vi "saveFuzzyMap2MCU.vi"(1 "Config":T1, 3 "error in (no error)":errorcluster) -> (10 "error out":errorcluster)   [LabVIEW 2016]
uses:
  Settings/Settings.ctl
  Logging/Logging Configuration.ctl
  Hardware Configuration.ctl
  <vilib>/NI Modbus.llb/MB Serial Master Query Write Multiple Registers (poly).vi
  Logging/Logging.lvlib
  Acquisition.lvlib
  Settings/Settings.lvlib
panel:
  out "Exception Code":u8 format="%.0x"
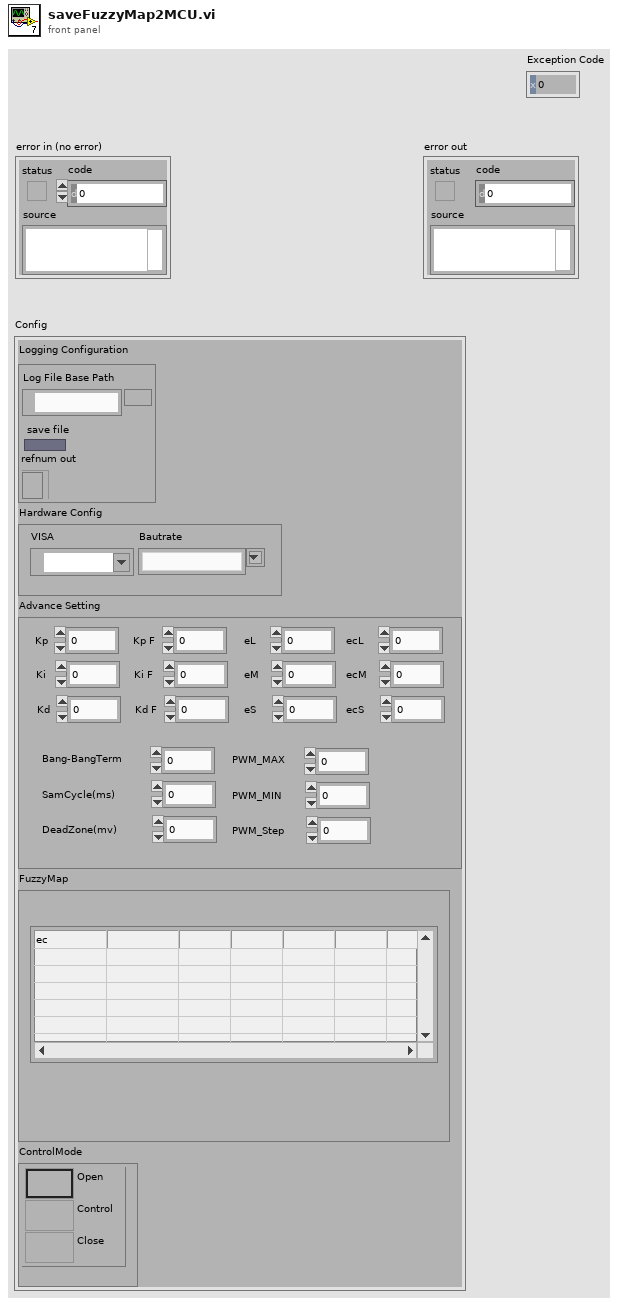
[diagram p1: front panel]
types:
  T1 = typedef "Settings.lvlib/Settings.ctl" = cluster{"Logging Configuration":T2, "Hardware Config":cluster{"Bautrate":string, "VISA":T3}, "Advance Setting":cluster{"PWM_Step":dbl, "PWM_MIN":dbl, "PWM_MAX":dbl, "DeadZone(mv)":dbl, "SamCycle(ms)":dbl, "Bang-BangTerm":dbl, "ecS":dbl, "ecM":dbl, "ecL":dbl, "eS":dbl, "eM":dbl, "eL":dbl, "Kd F":dbl, "Ki F":dbl, "Kp F":dbl, "Kd":dbl, "Ki":dbl, "Kp":dbl}, "FuzzyMap":cluster{"Table":string[][]}, "ControlMode":cluster{"Control":enum32{"1", "2", "4"}}}
  T2 = typedef "Logging.lvlib/Logging Configuration.ctl" = cluster{"Log File Base Path":path, "save file":bool, "refnum out":refnum<file>}
  T3 = typedef "Acquisition.lvlib/Hardware Configuration.ctl" = refnum<visa-resource-name>
  T4 = cluster{"Mode":enum16{"RTU", "ASCII"}, "Slave Address":u8}
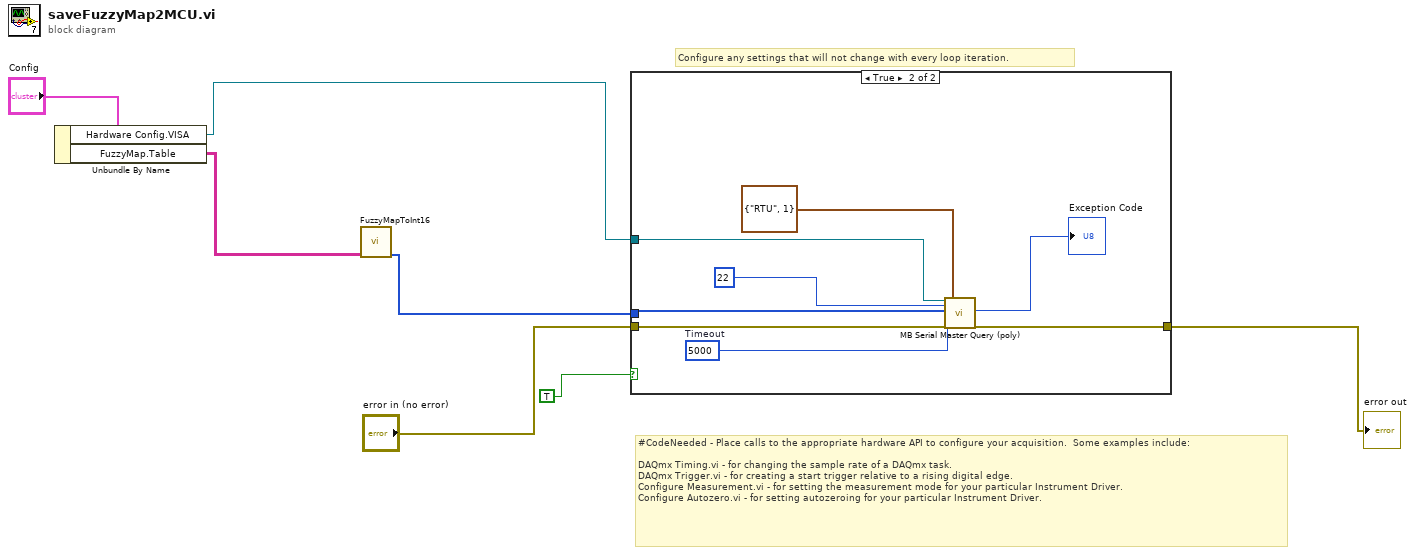
[diagram p0: block diagram]
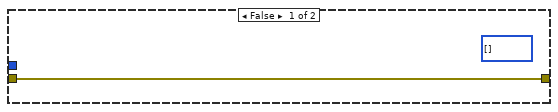
[diagram p2: hidden frame]
diagram:
  # "Configure any settings that will not change with every loop iteration."
  # "#CodeNeeded - Place calls to the appropriate hardware API to configure your acquisition.  Some examples include:\n\nDAQmx Timing.vi - for changing the sample rate of a DAQmx task.\nDAQmx Trigger.vi - for creating a start trigger relative to a rising digital edge.\nConfigure Measurement.vi - for setting the measurement mode for your particular Instrument Driver.\nConfigure Autozero.vi - for setting autozeroing for your particular Instrument Driver."
  n1 = Unbundle By Name("Config") -> ("Hardware Config.VISA"=w6:T3, "FuzzyMap.Table"=w2:string[][])
  n2 = call "FuzzyMapToInt16.vi"("Table Control"=w2) -> ("Array 2"=w1:u16[])  [unwired: 10 in]
  n3 = case shown="True" TRUE {
    tunnel: w6 -> [_ w16]
    tunnel: w1 -> [_ w11]
    tunnel: "error in (no error)" -> [w8 w10]
    tunnel: [w8 w9] -> w3
    frame False {
      (unwired) u16[] [] ("Input Registers")
    }
    frame True {
      w14 = u32 5000  # Timeout
      n4 = call-poly <vilib>:"MB Serial Master Query (poly).vi"("VISA resource name"=w16, "Starting Address"=u16 22, "Registers"=w11, "Timeout"=w14, "error in"=w10, "Serial Parameters"=T4 {"Mode"=enum."RTU", "Slave Address"=1}) -> ("Exception Code"=→"Exception Code":u8, "error out"=w9:errorcluster)  [unwired: 11 in, 1 out]
    }
  }
  "error out" <- w3
